vi "Control motion 2.vi"() -> ()   [LabVIEW 2019]
uses:
  <vilib>/robotics/Steering/Wheel/Wheel Parameters.ctl
  <vilib>/robotics/Steering/Wheel/Rotation Direction.ctl
  <vilib>/Analysis/coordinate.llb/2D Cartesian Coordinate Rotation.vi
  <vilib>/Analysis/coordinate.llb/2D Cartesian Coordinate Rotation (Scalar).vi
  <vilib>/robotics/Steering/Omnidirectional Wheel/NI_Robotics_Omnidirectional Wheel.lvclass
  C:/Program Files (x86)/National Instruments/LabVIEW 2019/vi.lib/robotics/Steering/Wheel/NI_Robotics_Wheel.lvclass
  <vilib>/robotics/Steering/Omnidirectional Wheel/Create Omnidirectional Wheel.vi
  <vilib>/robotics/Steering/Steering Frame/Create User Defined Steering Frame.vi
  <vilib>/robotics/Steering/Steering Frame/Apply Steering Frame Velocity to Motors.vi
  <vilib>/robotics/Steering/Steering Frame/Get Steering Frame Velocity from Motors.vi
  <vilib>/robotics/Steering/Wheel/NI_Robotics_Wheel.lvclass
  <vilib>/robotics/Steering/Steering Frame/NI_Robotics_Steering Frame.lvclass
panel:
  in  "Set Theta":dbl
  in  "Set Y":dbl
  in  "Set X":dbl
  out "Theta":dbl
  out "Y":dbl
  out "X":dbl
  in  "ccw motor angle states (rad)":dbl[](array[numeric])
  in  "ccw motor velocity states":dbl[](array[numeric])
  out "ccw motor angle setpoints (rad)":dbl[](array[numeric])
  out "ccw motor velocity setpoints":dbl[](array[numeric])
  in  "Velocity":T1(ring)=enum."Relative to Global Frame"
  in  "stop":bool
  out "complete":bool
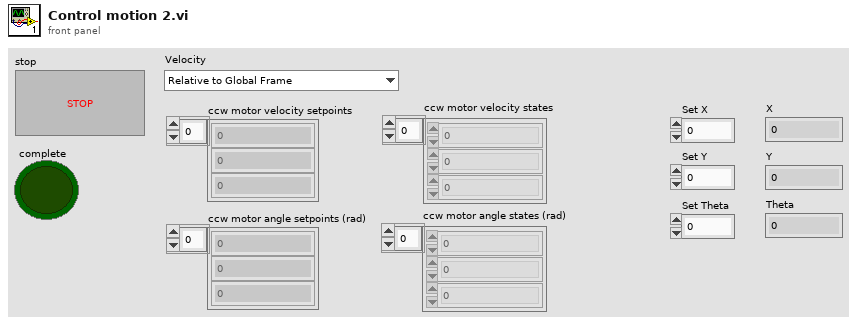
[diagram p1: front panel]
types:
  T1 = enum16{"Relative to Steering Frame", "Relative to Global Frame"}
  T2 = typedef "NI_Robotics_Wheel.lvclass/Rotation Direction.ctl" = u16
  T3 = typedef "NI_Robotics_Wheel.lvclass/Wheel Parameters.ctl" = cluster{"wheel radius":dbl, "gear ratio":dbl, "forward rotation direction":T2}
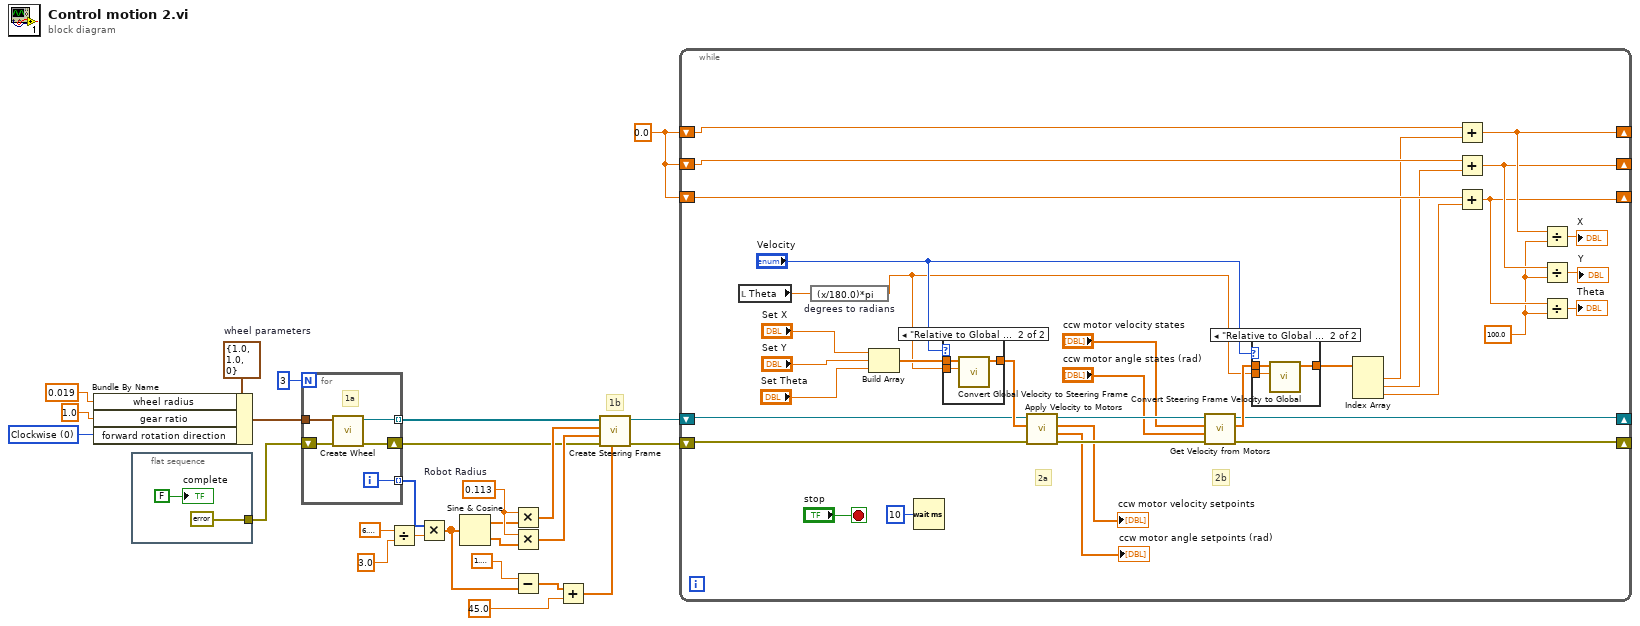
[diagram p0: block diagram]
diagram:
  w1 = 0.0
  w12 = T2 0 items=["Clockwise", "Counterclockwise"] ("forward rotation direction")
  w16 = 0.113  # Robot Radius
  w26 = T3 {"wheel radius"=1.0, "gear ratio"=1.0, "forward rotation direction"=0}  # wheel parameters
  # "1b"
  n1 = Bundle By Name(cluster=w26, "wheel radius"=0.019, "gear ratio"=1.0, "forward rotation direction"=w12) -> (w23:T3)
  n2 = flat-sequence {
    tunnel: [errorcluster {"status"=FALSE, "code"=0, "source"=""} ("error out")] -> w22
    frame #0 {
      "complete" <- FALSE ("complete")
    }
  }
  n3 = for {
    N: 3 -> [_]
    shift-right: [w32] -> w10
    shift-left: w22 -> [w33]
    tunnel: [w31] -> w21 mode=indexing
    tunnel: w23 -> [w30]
    tunnel: [w29] -> w17 mode=indexing
    i -> [w29]
    # "1a"
    n4 = call-poly <vilib>:"Create Wheel.vi"("error in (no error)"=w33, "wheel parameters"=w30) -> ("error out"=w32:errorcluster, "omni wheel out"=w31:refnum<class "NI_Robotics_Omnidirectional Wheel.lvclass">)  [unwired: 8 in]
  }
  n5 = Divide(x=6.283185307179586, y=3.0) -> (x/y=w18:dbl)
  n6 = Multiply(x=w17, y=w18) -> (x*y=w9:dbl[])
  n7 = Sine & Cosine(0:w9) -> (1:w8:dbl[], 2:w7:dbl[])
  n8 = Multiply(x=w16, y=w8) -> (x*y=w15:dbl[])
  n9 = Multiply(x=w16, y=w7) -> (x*y=w14:dbl[])
  n10 = Subtract(x=1.5707963267948966, y=w9) -> (x-y=w6:dbl[])
  n11 = Add(x=w6, y=45.0) -> (x+y=w5:dbl[])
  n12 = call-poly <vilib>:"Create Steering Frame.vi"("wheel frame angles (rad)"=w5, "error in (no error)"=w10, "wheel y positions"=w14, "wheel x positions"=w15, "wheels"=w21) -> ("error out"=w2:errorcluster, "steering frame out"=w3:refnum<class "NI_Robotics_Steering Frame.lvclass">)  [unwired: 5 in]
  n13 = while {
    shift-right: [w54] -> _
    shift-left: w3 -> [w59]
    shift-right: [w53] -> _
    shift-left: w2 -> [w58]
    shift-right: [w37] -> _
    shift-left: w1 -> [w50]
    shift-right: [w36] -> _
    shift-left: w1 -> [w49]
    shift-right: [w35] -> _
    shift-left: w1 -> [w48]
    stop <- "stop" stop-if-true
    w34 = 100.0 ("y")
    # "2b"
    # "2a"
    n14 = local read "Theta"() -> (w44:dbl)
    n15 = expression code="(x/180.0)*pi" "degrees to radians"(w44) -> (w60:dbl)
    n16 = Build Array("Set X", "Set Y", "Set Theta") -> (w64:dbl[])
    n17 = Wait (ms)(milliseconds to wait=u32 10) -> ()  [unwired: 1 out]
    n18 = case shown="\"Relative to Global Frame\"" "Velocity" {
      tunnel: w64 -> [w73 w76]
      tunnel: [w73 w75] -> w63
      tunnel: w60 -> [_ w74]
      frame "Relative to Steering Frame", Default {
      }
      frame "Relative to Global Frame" {
        n19 = call <vilib>:"Convert Global Velocity to Steering Frame.vi"("steering frame angle (rad)"=w74, "global velocity"=w76) -> ("steering frame velocity"=w75:dbl[])  [unwired: 9 in]
      }
    }
    n20 = call-poly <vilib>:"Apply Velocity to Motors.vi"("error in (no error)"=w58, "steering frame velocity"=w63, "steering frame in"=w59) -> ("error out"=w66:errorcluster, "ccw motor angle setpoints (rad)"=→"ccw motor angle setpoints (rad)":dbl[], "ccw motor velocity setpoints"=→"ccw motor velocity setpoints":dbl[], "steering frame out"=w67:refnum<class "NI_Robotics_Steering Frame.lvclass">)  [unwired: 4 in, 1 out]
    n21 = call-poly <vilib>:"Get Velocity from Motors.vi"("error in (no error)"=w66, "ccw motor angle states (rad)"="ccw motor angle states (rad)", "ccw motor velocity states"="ccw motor velocity states", "steering frame in"=w67) -> ("error out"=w53:errorcluster, "estimated steering frame velocity"=w62:dbl[], "steering frame out"=w54:refnum<class "NI_Robotics_Steering Frame.lvclass">)  [unwired: 5 in]
    n22 = case shown="\"Relative to Global Frame\"" "Velocity" {
      tunnel: w62 -> [w69 w72]
      tunnel: [w69 w71] -> w61
      tunnel: w60 -> [_ w70]
      frame "Relative to Steering Frame", Default {
      }
      frame "Relative to Global Frame" {
        n23 = call <vilib>:"Convert Steering Frame Velocity to Global.vi"("steering frame angle (rad)"=w70, "steering frame velocity"=w72) -> ("global velocity"=w71:dbl[])  [unwired: 9 in]
      }
    }
    n24 = Index Array(array=w61) -> (element #1=w47:dbl, element #2=w46:dbl, element #3=w45:dbl)  [unwired: 3 in]
    n25 = Add(x=w50, y=w47) -> (x+y=w37:dbl)
    n26 = Add(x=w49, y=w46) -> (x+y=w36:dbl)
    n27 = Add(x=w48, y=w45) -> (x+y=w35:dbl)
    n28 = Divide(x=w37, y=w34) -> (x/y=→"X":dbl)
    n29 = Divide(x=w36, y=w34) -> (x/y=→"Y":dbl)
    n30 = Divide(x=w35, y=w34) -> (x/y=→"Theta":dbl)
  }
